vi "Untitled 4 (SubVI).vi"(10 "Сколько битов брать":i32, 11 "Array in":dbl[](array[numeric])) -> (3 "Array out":dbl[](array[numeric]))   [LabVIEW 2017]
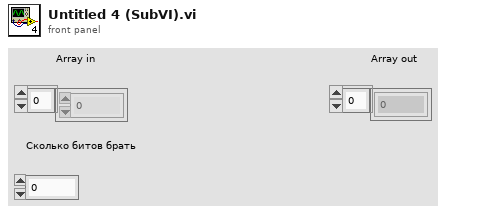
[diagram p1: front panel]
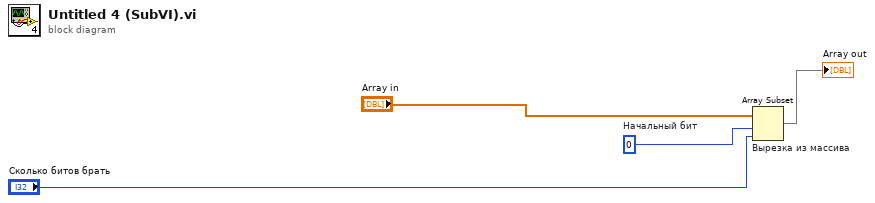
[diagram p0: block diagram]
diagram:
  w1 = 0  # Начальный бит
  n1 = Array Subset "Вырезка из массива"(array="Array in", index=w1, length="Сколько битов брать") -> (→"Array out":dbl[])
